vi "Incorrect PW (Max Attempts Reached).vi"(8 "error in (no error)":errorcluster) -> (0 "error out":errorcluster)   [LabVIEW 2021]
panel:
  # "Password was Incorrect or name characters < 4\nYou have breached the maximum number of Log In attempts.\nThis application will now shut down"
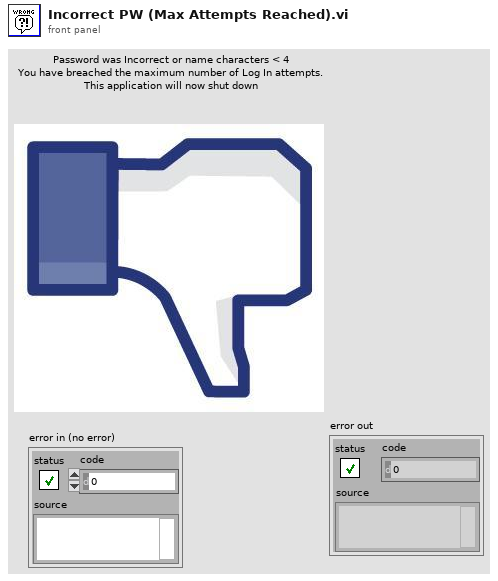
[diagram p1: front panel]
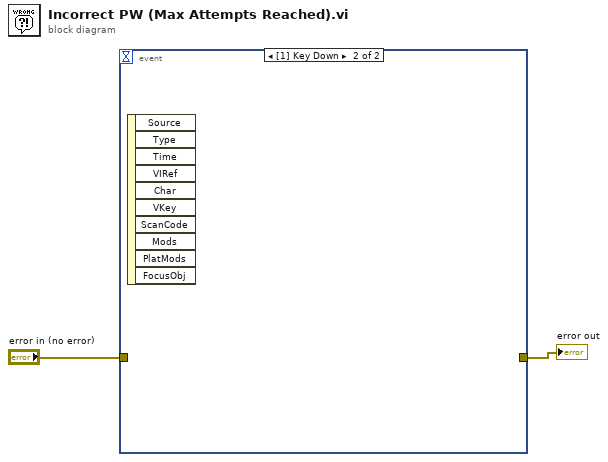
[diagram p0: block diagram]
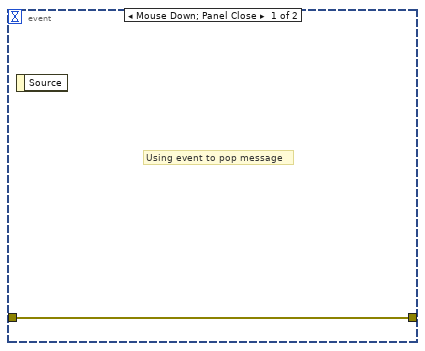
[diagram p2: hidden frame]
diagram:
  n1 = event shown="[1] Key Down" {
    selector: _ -> [_ _]
    dyn-events: _ -> [_ _]
    timeout: _ -> [_ _]
    tunnel: "error in (no error)" -> [w3 _]
    tunnel: [w3 _] -> w1
    event Mouse Down; Panel Close {
      # "Using event to pop message"
      n2 = event-data() -> ()  [unwired: 1 in, 1 out]
    }
    event Key Down {
      n3 = event-data() -> ()  [unwired: 1 in, 10 out]
    }
  }
  "error out" <- w1
